vi "MainNR.vi"(10 "JQMHStartup":refnum<class "ModuleStartup.lvclass">, 11 "NewTemplate in":refnum<class "TitleBar.lvclass">) -> ()   [LabVIEW 2024, in "TitleBar.lvclass"]
uses:
  TitleBar.lvclass
  TitleBar.lvclass/TitleBar.ctl
  C:/Git/JA/JQMH/RQMHCore/ModuleCore/Module.lvclass
  C:/Git/JA/JQMH/ModuleTemplates/TitleBar/TitleBar.lvclass
  RQMHCore/ModuleCore/Module.lvclass
  RQMHCore/Startup/ModuleStartup.lvclass
  RQMHCore/ModQueue/ModuleQueue.lvclass
  RQMHCore/Shared/ModuleShared.lvlib
  RQMHCore/ModuleCore/InitialiseReplyArgs.ctl
  Do Something Args.ctl
  Do Something ReplyArgs.ctl
  user32.dll
  RQMHCore/ModQueue/Delacor_lib_QMH_Enqueue Message (Single).vi
  AddTopLevelVI Args.ctl
  AddTopLevelVI ReplyArgs.ctl
panel:
  out "String":string
  out "error out":errorcluster
  in  "Minimise":bool
  in  "Maximise":bool
  in  "Close":bool
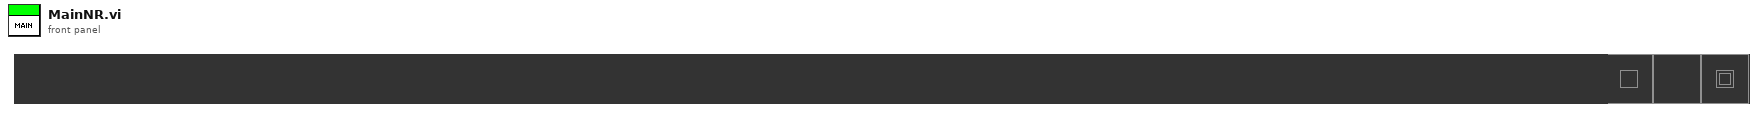
[diagram p1: front panel]
types:
  T1 = typedef "TitleBar.lvclass/Request Events--cluster.ctl" = cluster{"Do Something":refnum<user-event>, "AddTopLevelVI":refnum<user-event>}
  T2 = cluster{"Stop Module":refnum<user-event>, "Requests":T1}
  T3 = enum32{"Invalid", "Standard", "Closed", "Hidden", "Minimized", "Maximized"}
  T4 = typedef "Module.lvclass/InitialiseReplyArgs.ctl" = cluster{"Did Init?":bool}
  T5 = typedef "TitleBar.lvclass/Do Something Args.ctl" = cluster{"Msg":string}
  T6 = typedef "TitleBar.lvclass/Do Something ReplyArgs.ctl" = cluster{"Value":dbl, "Boolean":bool}
  T7 = typedef "TitleBar.lvclass/AddTopLevelVI Args.ctl" = cluster{"MainRef":refnum<vi>}
  T8 = typedef "TitleBar.lvclass/AddTopLevelVI ReplyArgs.ctl" = cluster{"null":bool}
  T9 = typedef "Module.lvclass/Reply.ctl" = cluster{"Expects Reply":bool, "Reply":refnum<notifier>}
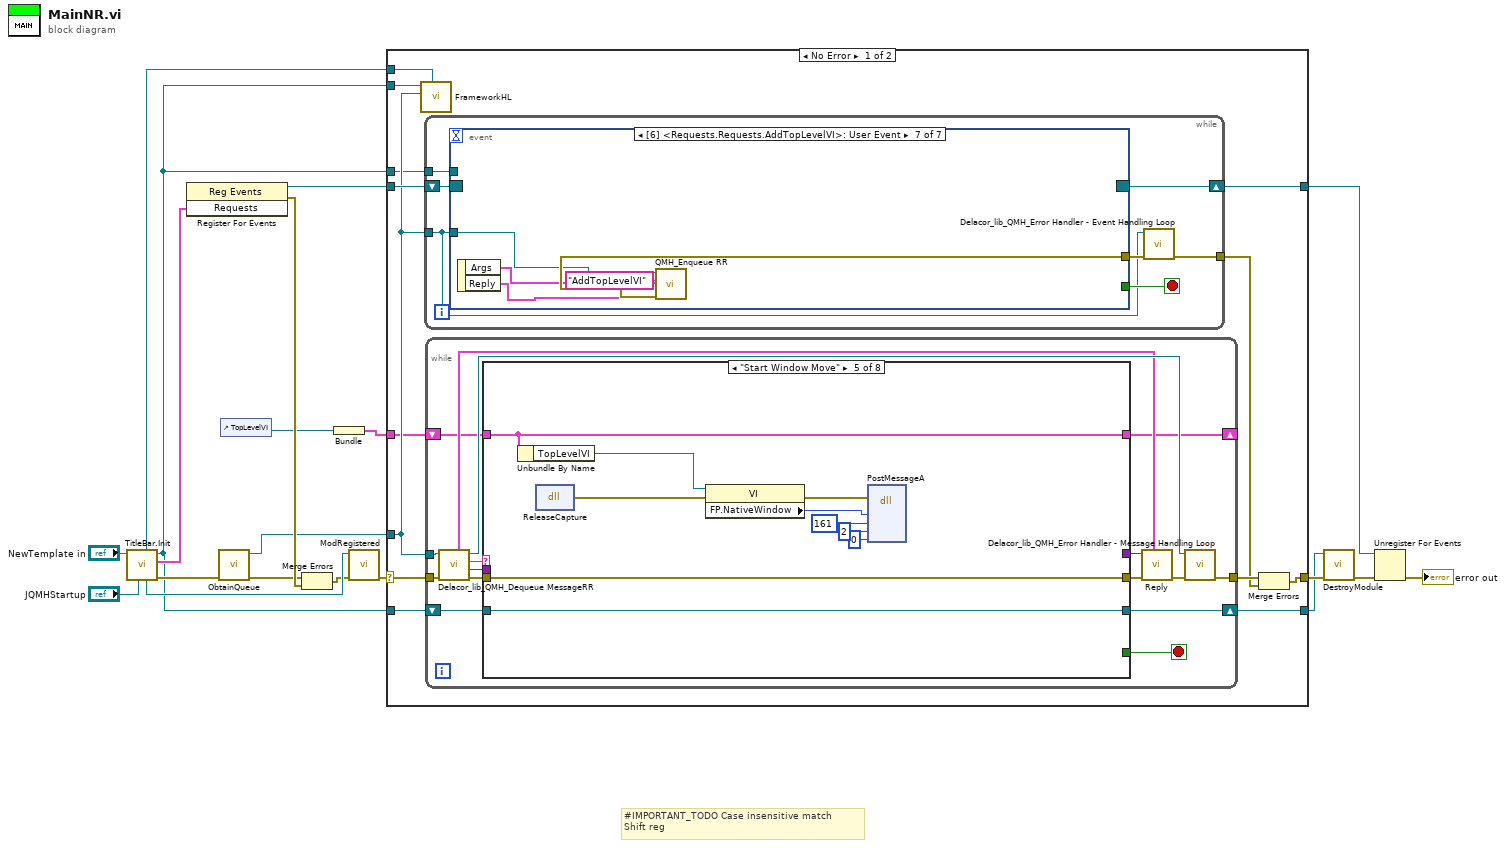
[diagram p0: block diagram]
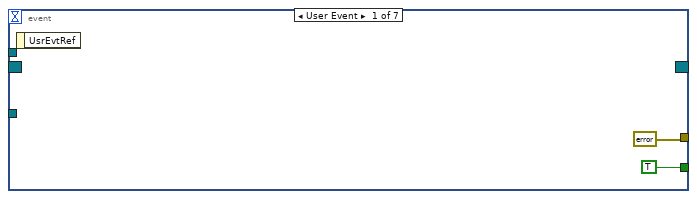
[diagram p2: hidden frame]
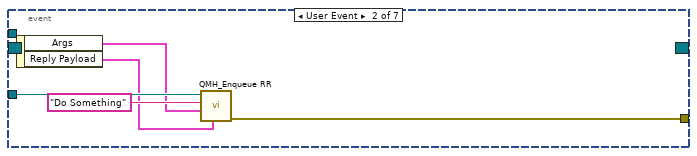
[diagram p3: hidden frame]
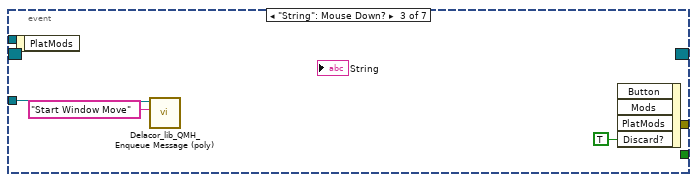
[diagram p4: hidden frame]
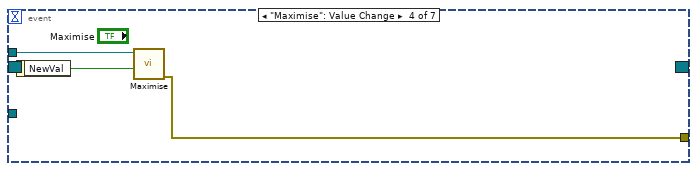
[diagram p5: hidden frame]
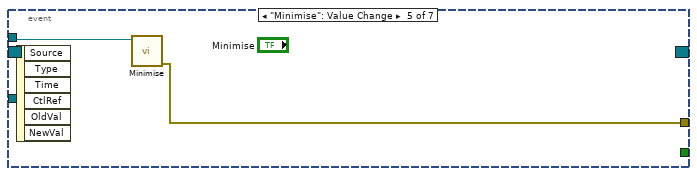
[diagram p6: hidden frame]
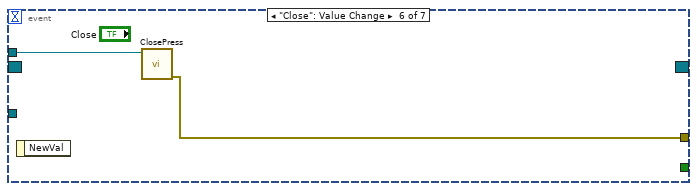
[diagram p7: hidden frame]
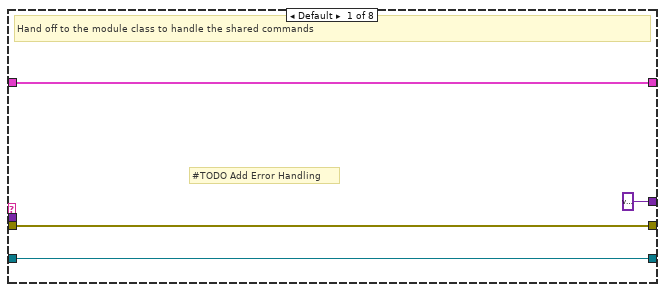
[diagram p8: hidden frame]
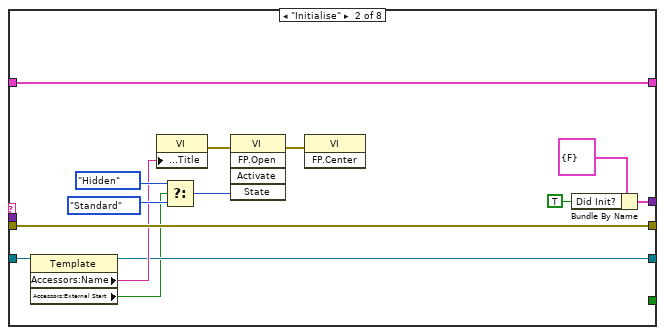
[diagram p9: hidden frame]
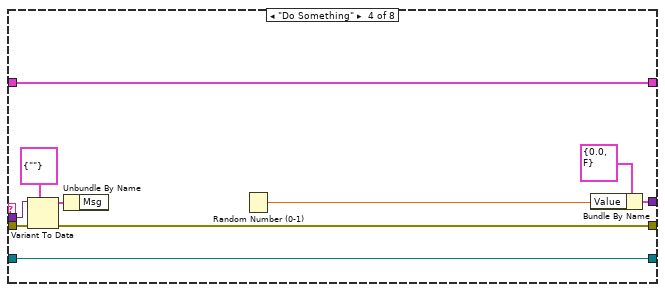
[diagram p11: hidden frame]
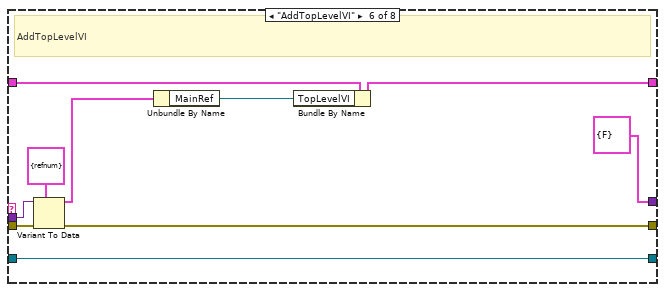
[diagram p12: hidden frame]
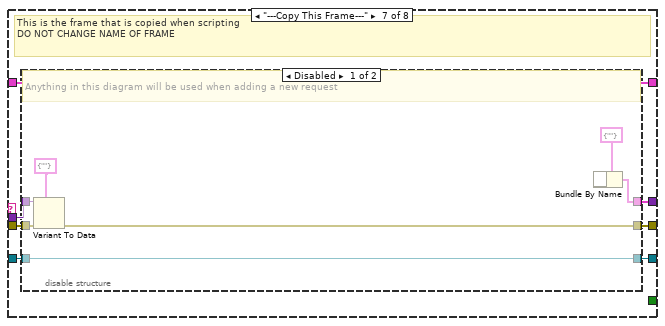
[diagram p13: hidden frame]
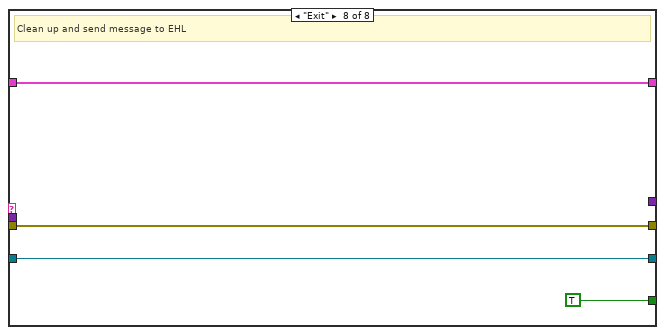
[diagram p15: hidden frame]
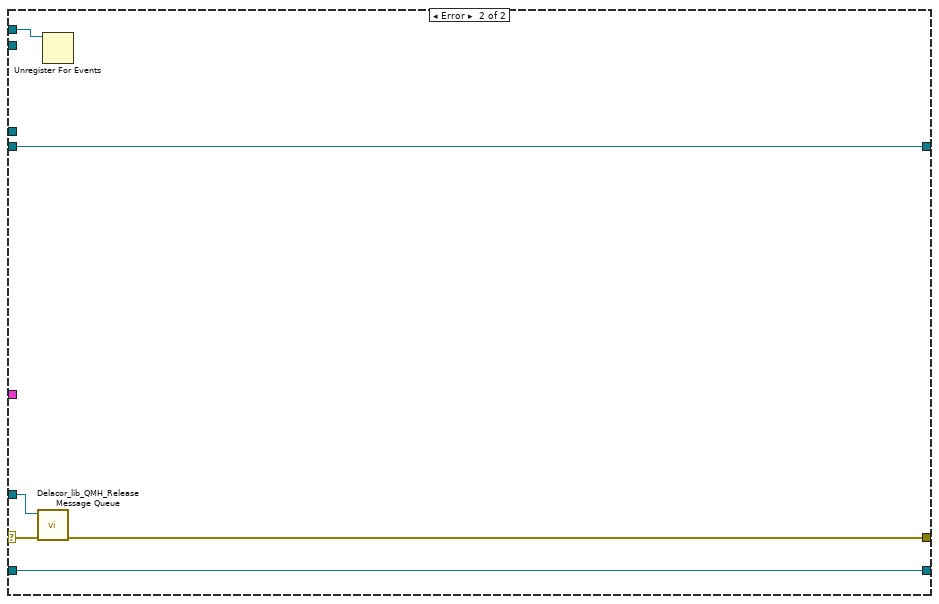
[diagram p16: hidden frame]
diagram:
  # "#IMPORTANT_TODO Case insensitive match\nShift reg"
  n1 = call "TitleBar.Init.vi"("JQMHStartup in"="JQMHStartup", "NewTemplate in"="NewTemplate in") -> ("error out"=w13:errorcluster, "Requests"=w4:T2, "NewTemplate out"=w3:refnum<class "TitleBar.lvclass">, "JQMHStartup out"=w11:refnum<class "ModuleStartup.lvclass">, "StandardRequests"=w7:refnum<event-registration>)  [unwired: 4 in, 1 out]
  n2 = register-events(w4) -> (reference out=w6:refnum<event-registration>, error out=w20:errorcluster)  [unwired: 2 in]
  n3 = call "ObtainQueue.vi"("error in"=w13) -> ("error out"=w12:errorcluster, "Message Queue"=w8:refnum<class "ModuleQueue.lvclass">)  [unwired: 9 in]
  n4 = control-ref of="TopLevelVI"() -> (w2:refnum<vi>)
  n5 = Merge Errors(w12, w20) -> (w9:errorcluster)
  n6 = Bundle("TopLevelVI"=w2) -> (w1:cluster{"TopLevelVI":refnum<vi>})  [unwired: 1 in]
  n7 = call "ModRegistered.vi"("error in (no error)"=w9, "JQMHStartup in"=w11) -> ("error out"=w10:errorcluster)  [unwired: 9 in]
  n8 = case "RQMH_MAIN" shown="No Error" w10 {
    selector: w10 -> [w30 w153]
    tunnel: w3 -> [w33 w152]
    tunnel: [w32 w155] -> w19
    tunnel: w6 -> [w31 w155]
    tunnel: w8 -> [w24 w154]
    tunnel: [w29 w152] -> w5
    tunnel: [w26 w151] -> w16
    tunnel: w3 -> [w25 _]
    tunnel: w7 -> [w23 w150]
    tunnel: w3 -> [w22 _]
    tunnel: w1 -> [w21 _]
    frame No Error {
      n9 = call-dynamic "FrameworkHL.vi"("StandardRequests"=w23, "Message Queue"=w24, "JQMHModule in"=w25) -> ()  [unwired: 9 in]
      n10 = while {
        shift-right: [w40] -> w32
        shift-left: w31 -> [w35]
        tunnel: w24 -> [w36]
        tunnel: [w37] -> w27
        tunnel: w22 -> [w34]
        stop <- w39 stop-if-true
        n11 = event "RQMH_EVENT_MAIN" shown="[6] <Requests.Requests.AddTopLevelVI>: User Event" {
          selector: w35 -> [_ _ _ _ _ _ _]
          dyn-events: [_ _ _ _ _ _ _] -> w40
          timeout: _ -> [_ _ _ _ _ _ _]
          tunnel: [TRUE _ _ _ _ _ _] -> w39
          tunnel: w36 -> [_ w47 w49 _ _ _ w59]
          tunnel: [errorcluster {"status"=FALSE, "code"=0, "source"=""} ("error out") w44 _ w51 w54 w56 w62] -> w38
          tunnel: w34 -> [_ _ _ w52 w55 w57 _]
          event User Event {
            n12 = event-data() -> ()  [unwired: 1 in, 1 out]
          }
          event User Event {
            n13 = event-data() -> ("Args"=w45:T5, "Reply Payload"=w43:T9)  [unwired: 1 in]
            n14 = call "QMH_Enqueue RR.vi"("Reply"=w43, "Message Data"=w45, "Message"="Do Something", "Message Queue in"=w47) -> ("error out"=w44:errorcluster)  [unwired: 6 in, 1 out]
          }
          event "String": Mouse Down? {
            n15 = event-data() -> ()  [unwired: 1 in, 1 out]
            n16 = call-poly "Delacor_lib_QMH_Enqueue Message (poly).vi"("Message"="Start Window Move", "Message Queue in"=w49) -> ()  [unwired: 8 in, 2 out]
            n17 = event-data("Discard?"=TRUE) -> ()  [unwired: 4 in, 1 out]
          }
          event "Maximise": Value Change {
            n18 = event-data() -> ("NewVal"=w53:bool)  [unwired: 1 in]
            n19 = call "Maximise.vi"("Maximised"=w53, "module in"=w52) -> ("error out"=w51:errorcluster)  [unwired: 8 in, 1 out]
          }
          event "Minimise": Value Change {
            n20 = event-data() -> ()  [unwired: 1 in, 6 out]
            n21 = call "Minimise.vi"("module in"=w55) -> ("error out"=w54:errorcluster)  [unwired: 9 in, 1 out]
          }
          event "Close": Value Change {
            n22 = event-data() -> ()  [unwired: 1 in, 1 out]
            n23 = call "ClosePress.vi"("module in"=w57) -> ("error out"=w56:errorcluster)  [unwired: 9 in, 1 out]
          }
          event User Event {
            n24 = event-data() -> ("Args"=w60:T7, "Reply"=w61:T9)  [unwired: 1 in]
            n25 = call "QMH_Enqueue RR.vi"("Reply"=w61, "Message Data"=w60, "Message"="AddTopLevelVI", "Message Queue in"=w59) -> ("error out"=w62:errorcluster)  [unwired: 6 in, 1 out]
          }
        }
        n26 = call-dynamic "Delacor_lib_QMH_Error Handler - Event Handling Loop.vi"("error in"=w38, "Message Queue in"=w36) -> ("dup error in"=w37:errorcluster)  [unwired: 8 in, 1 out]
      }
      n27 = while {
        tunnel: w24 -> [w73]
        tunnel: w30 -> [w72]
        shift-right: [w75] -> w29
        shift-left: w33 -> [w76]
        tunnel: [w74] -> w28
        shift-right: [w63] -> _
        shift-left: w21 -> [w64]
        stop <- w78 stop-if-true
        n28 = call-dynamic "Delacor_lib_QMH_Dequeue MessageRR.vi"("error in"=w72, "Message Queue in"=w73) -> ("error out"=w71:errorcluster, "Message Data"=w69:variant, "Message"=w70:string, "Message Queue out"=w77:refnum<class "ModuleQueue.lvclass">, "Reply"=w65:T9)  [unwired: 5 in]
        n29 = case "RQMH_MESSAGE_CASES" shown="\"Start Window Move\"" w70 {
          tunnel: [_ _ _ _ _ _ _ TRUE] -> w78
          tunnel: w76 -> [w81 w85 w98 w109 w118 w127 w134 w148]
          tunnel: w69 -> [_ _ _ w105 _ w126 w132 _]
          tunnel: w71 -> [w82 w96 w99 w104 w119 w129 w136 w147]
          tunnel: [w82 w96 w99 w103 w119 w128 w135 w147] -> w68
          tunnel: [w81 w86 w98 w109 w118 w127 w133 w148] -> w75
          tunnel: [variant w95 _ w108 _ T8 {"null"=FALSE} ("RQMH_MHL_REPLY_PL") w131 _] -> w66
          tunnel: w64 -> [w79 w83 w97 w100 w111 w123 w130 w146]
          tunnel: [w79 w83 w97 w100 w111 w122 w130 w146] -> w63
          frame Default {
            # "#TODO Add Error Handling"
            # "Hand off to the module class to handle the shared commands"
          }
          frame "Initialise" {
            n30 = property class="Template"(reference=w85) -> (reference out=w86:refnum<class "TitleBar.lvclass">, "Accessors:Name"=w87:string, "Accessors:External Start"=w84:bool)  [unwired: 1 in, 1 out]
            n31 = property on="Property Node" class="VI"("Front Panel.Title"=w87) -> (error out=w93:errorcluster)  [unwired: 2 in, 1 out]
            n32 = Select(t=T3."Hidden" ("State"), s=w84, f=T3."Standard" ("State")) -> (s? t:f=w89:T3)
            n33 = invoke on="Invoke Node" class="VI" method="FP.Open"(error in=w93, "State"=w89) -> (error out=w92:errorcluster)  [unwired: 3 in, 4 out]
            n34 = invoke on="Invoke Node" class="VI" method="FP.Center"(error in=w92) -> ()  [unwired: 2 in, 3 out]
            n35 = Bundle By Name(cluster=T4 {"Did Init?"=FALSE} ("Args"), "Did Init?"=TRUE) -> (w95:T4)
          }
          frame "---Module Specific---" {
          }
          frame "Do Something" {
            n36 = Variant To Data(error in=w104, type=T5 {"Msg"=""} ("Do Something Args"), Variant=w105) -> (data=w101:T5, error out=w103:errorcluster)
            n37 = Unbundle By Name(w101) -> ()  [unwired: 1 out]
            n38 = Random Number (0-1)() -> (number: 0 to 1=w106:dbl)
            n39 = Bundle By Name(cluster=T6 {"Value"=0.0, "Boolean"=FALSE}, "Value"=w106) -> (w108:T6)
          }
          frame "Start Window Move" {
            n40 = Unbundle By Name(w111) -> ("TopLevelVI"=w110:refnum<vi>)
            n41 = dll-call lib="user32.dll" fn="ReleaseCapture"() -> (error out=w117:errorcluster)  [unwired: 4 in, 1 out]
            n42 = property class="VI"(reference=w110, error in=w117) -> (error out=w116:errorcluster, "FP.NativeWindow"=w115:u64)  [unwired: 1 out]
            n43 = dll-call lib="user32.dll" fn="PostMessageA"(error in=w116, "hWnd"=w115, "Msg"=161, "wParam"=2, "lParam"=0) -> ()  [unwired: 7 in, 2 out]
          }
          frame "AddTopLevelVI" {
            # "AddTopLevelVI"
            n44 = Variant To Data(error in=w129, type=T7 {"MainRef"=refnum} ("RQMH_MHL_MSG_PL"), Variant=w126) -> (data=w121:T7, error out=w128:errorcluster)
            n45 = Unbundle By Name(w121) -> ("MainRef"=w120:refnum<vi>)
            n46 = Bundle By Name(cluster=w123, "TopLevelVI"=w120) -> (w122:cluster{"TopLevelVI":refnum<vi>})
          }
          frame "---Copy This Frame---" {
            # "This is the frame that is copied when scripting\nDO NOT CHANGE NAME OF FRAME"
            n47 = disable-structure shown="Disabled" {
              disable-tunnel: w136 -> [w140 w145]
              disable-tunnel: [w141 w145] -> w135
              disable-tunnel: w134 -> [w143 w144]
              disable-tunnel: [w143 w144] -> w133
              disable-tunnel: w132 -> [w142 _]
              disable-tunnel: [w138 _] -> w131
              frame Disabled {
                # "Anything in this diagram will be used when adding a new request"
                n48 = Variant To Data(error in=w140, type=cluster{string} {""} ("RQMH_MHL_MSG_PL"), Variant=w142) -> (error out=w141:errorcluster)  [unwired: 1 out]
                n49 = Bundle By Name(cluster=cluster{string} {""} ("RQMH_MHL_REPLY_PL")) -> (w138:cluster{string})  [unwired: 1 in]
              }
              frame Enabled {
              }
            }
          }
          frame "Exit" {
            # "Clean up and send message to EHL"
          }
        }
        n50 = call "Reply.vi"("Reply"=w65, "error in (no error)"=w68, "ReplyPayload"=w66) -> ("error out"=w67:errorcluster)  [unwired: 8 in]
        n51 = call-dynamic "Delacor_lib_QMH_Error Handler - Message Handling Loop.vi"("error in"=w67, "Message Queue in"=w77) -> ("dup error in"=w74:errorcluster)  [unwired: 8 in, 1 out]
      }
      n52 = Merge Errors(w28, w27) -> (w26:errorcluster)
    }
    frame Error {
      n53 = call-dynamic "Delacor_lib_QMH_Release Message Queue.vi"("error in"=w153, "Message Queue"=w154) -> ("error out"=w151:errorcluster)  [unwired: 9 in]
      n54 = Unregister For Events(event registration refnum=w150) -> ()  [unwired: 1 in, 1 out]
    }
  }
  n55 = call "DestroyModule.vi"("error in (no error)"=w16, "JQMHModule in"=w5) -> ("error out"=w18:errorcluster)  [unwired: 9 in]
  n56 = Unregister For Events(event registration refnum=w19, error in=w18) -> (error out=→"error out":errorcluster)
